vi "TopRightHaveSameStone.vi"(0 "Row in":i32, 1 "StoneColor":u16, 5 "Col in":i32, 7 "Chessboard":T1, 9 "TatgetIndex":T2, 11 "error in (no error)":errorcluster) -> (3 "HaveSameStone?":bool, 4 "Row out":i32, 6 "Col out":i32, 8 "Chessboard out":T1, 10 "SSIndex":T2, 15 "error out":errorcluster)   [LabVIEW 2009]
doc: "To seek same stone in the TopRight direction.\n--------------------------------------------\nStoneColor: Witch stone type is seeking for.\nRow in: Start index number(Row).\nCol in: Start index number(Col).\nChessboard: The Chessboard seeking on.\nTargetIndex: Index mumber the seeking ends.\nHaveSameStone: If there are same stones this indicator returns TRUE.\nRow out: Pass out the start index number(Row).\nCol out: Pass out the start index number(Col).\nChessboard out: Pass out the Chessboard seeking on.\nSSIndex: Return the Index numbers of same stone."
uses:
  Controls/Chess.ctl
  Controls/ItemIndex.ctl
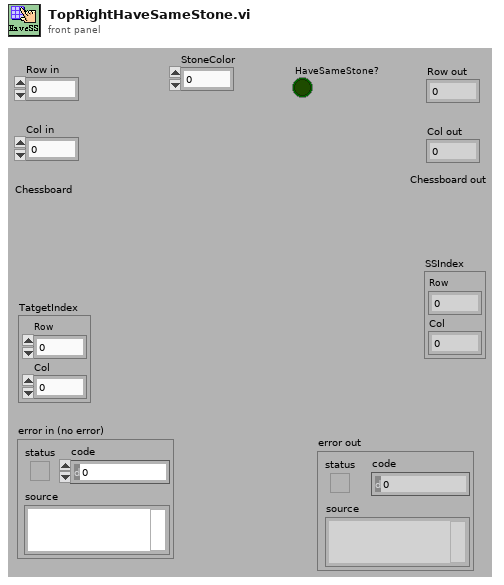
[diagram p1: front panel]
types:
  T1 = typedef "Chess.ctl" = u16[][]
  T2 = typedef "ItemIndex.ctl" = cluster{"Row":i32, "Col":i32}
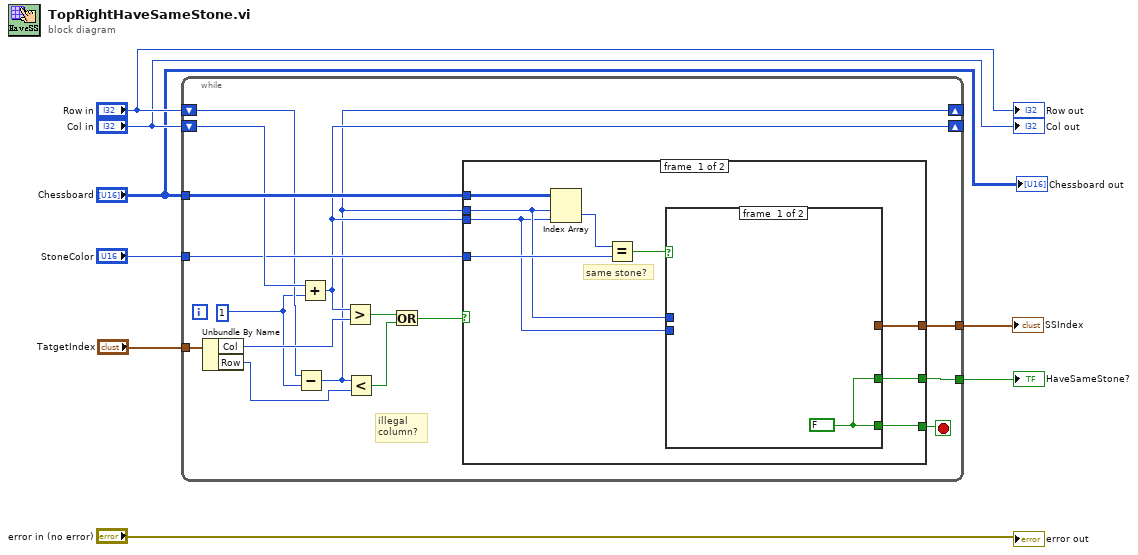
[diagram p0: block diagram]
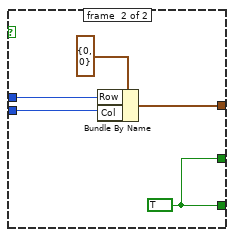
[diagram p2: hidden frame]
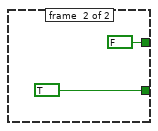
[diagram p3: hidden frame]
diagram:
  n1 = while {
    tunnel: "Chessboard" -> [w23]
    tunnel: "StoneColor" -> [w21]
    shift-right: [w10] -> _
    shift-left: "Row in" -> [w15]
    shift-right: [w17] -> _
    shift-left: "Col in" -> [w22]
    tunnel: [w20] -> w8
    tunnel: [w19] -> w5
    tunnel: "TatgetIndex" -> [w18]
    stop <- w24 stop-if-true
    w9 = 1 ("y")
    # "illegal \ncolumn?"
    n2 = Unbundle By Name(w18) -> ("Col"=w16:i32, "Row"=w14:i32)
    n3 = Subtract(x=w15, y=w9) -> (x-y=w10:i32)
    n4 = Add(x=w22, y=w9) -> (x+y=w17:i32)
    n5 = Greater?(x=w17, y=w16) -> (0:w13:bool)
    n6 = Less?(x=w10, y=w14) -> (x < y?=w12:bool)
    n7 = Or(x=w13, y=w12) -> (x .or. y?=w11:bool)
    n8 = case shown="True" w11 {
      tunnel: [w30 TRUE] -> w24
      tunnel: w23 -> [w33 _]
      tunnel: w17 -> [w26 _]
      tunnel: w10 -> [w27 _]
      tunnel: w21 -> [w29 _]
      tunnel: [w28 FALSE] -> w20
      tunnel: [w25 _] -> w19
      frame #0 {
        # "same stone?"
        n9 = Index Array(array=w33, index (row)=w27, index (col)=w26) -> (element=w32:u16)
        n10 = Equal?(x=w32, y=w29) -> (x = y?=w31:bool)
        n11 = case shown="True" w31 {
          tunnel: [w34 w39] -> w30
          tunnel: [w34 w39] -> w28
          tunnel: w27 -> [_ w37]
          tunnel: w26 -> [_ w36]
          tunnel: [_ w35] -> w25
          frame #0 {
            w34 = FALSE
          }
          frame #1 {
            w39 = TRUE
            n12 = Bundle By Name(cluster=T2 {"Row"=0, "Col"=0} ("ItemIndex"), "Row"=w37, "Col"=w36) -> (w35:T2)
          }
        }
      }
      frame #1 {
      }
    }
  }
  "HaveSameStone?" <- w8
  "SSIndex" <- w5
  "Col out" <- "Col in"
  "Row out" <- "Row in"
  "error out" <- "error in (no error)"
  "Chessboard out" <- "Chessboard"
